vi "Temperature Limit.vi"() -> ()   [LabVIEW 2015]
doc: "This VI simulates the acquisition of temperature, graphs the temperature, and notifies the user if the temperature is over the limit."
panel:
  in  "Start":bool
  in  "Delta t (ms)":i32(slide)=400 scale=50.0..500.0
  in  "Stop":bool
  in  "High Limit":dbl=28.0 format="%.2f"
  out "Temperature":cluster{"Temperature":dbl, "High Limit":dbl}(graph)={"Temperature"=85.88749999999999, "High Limit"=80.0}
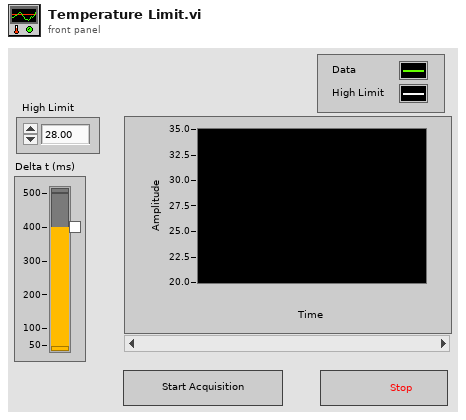
[diagram p1: front panel]
types:
  T1 = enum16{"Always On", "Always Off", "Off While Running"}
  T2 = cluster{"Temperature Value":dbl, "High Limit":dbl}
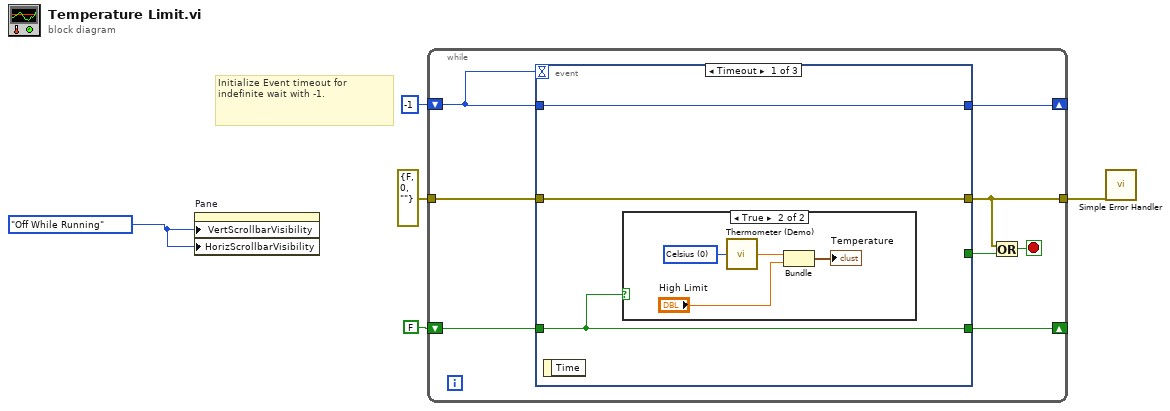
[diagram p0: block diagram]
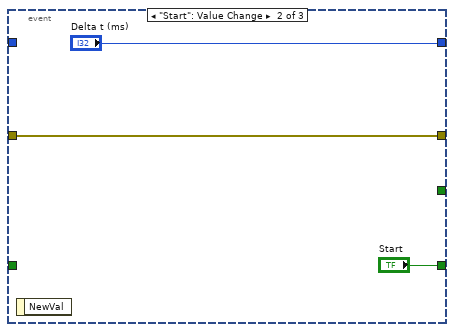
[diagram p3: hidden frame]
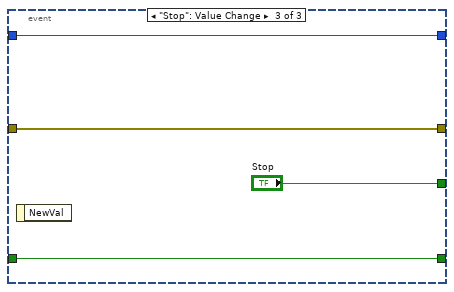
[diagram p4: hidden frame]
diagram:
  w1 = T1."Off While Running" ("Vertical Scrollbar Visibility")
  # "Initialize Event timeout for indefinite wait with -1."
  n1 = property on="Pane" class="Pane"("VertScrollbarVisibility"=w1, "HorizScrollbarVisibility"=w1) -> ()  [unwired: 2 in, 2 out]
  n2 = while {
    tunnel: errorcluster {"status"=FALSE, "code"=0, "source"=""} ("error out") -> [w13]
    tunnel: [w11] -> w4
    shift-right: [w9] -> _
    shift-left: FALSE ("Start") -> [w8]
    shift-right: [w7] -> _
    shift-left: -1 ("Delta t (ms)") -> [w6]
    stop <- w12 stop-if-true
    n3 = event shown="[0] Timeout" {
      selector: _ -> [_ _ _]
      dyn-events: _ -> [_ _ _]
      timeout: w6 -> [_ _ _]
      tunnel: [_ _ "Stop"] -> w10
      tunnel: w13 -> [w16 w21 w26]
      tunnel: [w16 w21 w26] -> w11
      tunnel: [w14 "Start" w25] -> w9
      tunnel: w8 -> [w14 _ w25]
      tunnel: [w15 "Delta t (ms)" w24] -> w7
      tunnel: w6 -> [w15 _ w24]
      event Timeout {
        n4 = event-data() -> ()  [unwired: 1 in, 1 out]
        n5 = case shown="True" w14 {
          frame False {
          }
          frame True {
            w17 = u16 0 items=["Celsius", "Fahrenheit"] ("Units (0: Celsius)")
            n6 = call "Thermometer (Demo).vi"("Units (0: Celsius)"=w17) -> ("Temperature Value"=w18:dbl)
            n7 = Bundle("Temperature Value"=w18, "High Limit"="High Limit") -> (→"Temperature":T2)  [unwired: 1 in]
          }
        }
      }
      event "Start": Value Change {
        n8 = event-data() -> ()  [unwired: 1 in, 1 out]
      }
      event "Stop": Value Change {
        n9 = event-data() -> ()  [unwired: 1 in, 1 out]
      }
    }
    n10 = Or(x=w11, y=w10) -> (x .or. y?=w12:bool)
  }
  n11 = call <vilib>:"Simple Error Handler.vi"("error in (no error)"=w4) -> ()  [unwired: 4 in, 5 out]
